vi "PPG_ABCGUI.panel.vi"() -> ()   [LabVIEW 2014, in "PPG_ABCGUI.lvlib"]
doc: "GUI to configure the FPGA card\n\nauthor: Dennis Neidherr, GSI\nlicense: GPL"
uses:
  PPG_ABCGUI.lvlib
  CSlibraries-extern/DimLVEvent/DimIndicators/DimIndicators.numericType.ctl
  CSlibraries-extern/DimLVEvent/DimIndicators/DimIndicators.anyType.ctl
  <vilib>/Utility/config.llb/Write Key (String).vi
  <vilib>/Utility/config.llb/Read Key (String).vi
  CSCore/CSSystem/CoreLib/CoreLib.int 2 byte array.vi
  CSCore/CSSystem/CoreLib/CoreLib.string 2 byte array.vi
  CSCore/CSSystem/CoreLib/CoreLib.double array 2 byte array.vi
  CSCore/CSSystem/CoreLib/CoreLib.lvlib
  CSCore/CSObj/CSObj.lvlib
  CSlibraries/UtilityLib/UtilityLib.lvlib
  CSCore/GUIs/GOGUserGUIs/DeviceBaseGUI/DeviceBaseGUI.lvlib
  CSlibraries-extern/DimLVEvent/DimIndicators/DimIndicators.lvlib
  CSCore/CSApplicationBaseClasses/DeviceBase/DeviceBase.lvlib
  CSCore/BaseProcess/BaseProcess.lvlib
  <vilib>/Utility/config.llb/NI_LVConfig.lvlib
panel:
  in  "Start":bool
  in  "SaveABC to File":bool
  in  "LoadABC from File":bool
  in  "LoadABC":bool
  out "FPGA state string":string
  in  "FPGA state":T1 caption="dic_service_numeric"
  in  "Outputs":string[][](table)
  in  "Timing":string[][](table)=[[""]]
  out "Busy":bool
  out "ErrorString":string
  out "deviceIDString":string
  out "loop counter":i32
  out "error out":errorcluster
  in  "error in (no error)":errorcluster
  in  "object ref":refnum<vi>
  in  "state":T1 caption="dic_service_numeric"
  in  "deviceID":T2 caption="dic_service_anyType"
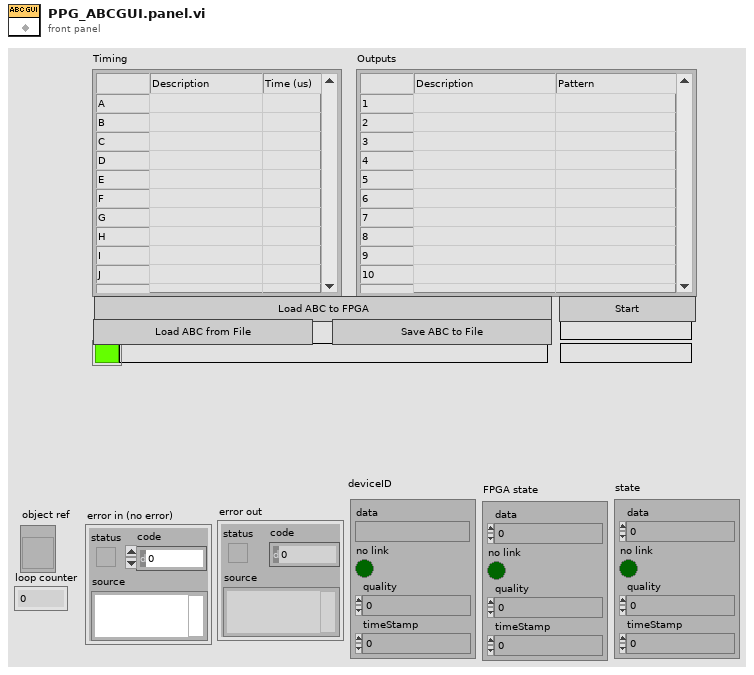
[diagram p1: front panel]
types:
  T1 = typedef "DimIndicators.lvlib/DimIndicators.numericType.ctl" = cluster{"data":dbl, "no link":bool, "quality":i32, "timeStamp":dbl}
  T2 = typedef "DimIndicators.lvlib/DimIndicators.anyType.ctl" = cluster{"data":string, "no link":bool, "quality":i32, "timeStamp":dbl}
  T3 = typedef "DeviceBaseGUI.lvlib/DeviceBaseGUI.i attribute.ctl" = cluster{"GOGFrontPanel.i attribute":T4}
  T4 = typedef "GOGFrontPanel.lvlib/GOGFrontPanel.i attribute.ctl" = cluster{"GOGObject":string, "Object":string, "Method":string, "Descriptor":T5, "Input Descriptor":string, "Output Descriptor":string, "inputNames":string[], "outputNames":string[], "Values":cluster{"descriptor":string, "value":string}[]}
  T5 = typedef "BaseProcess.lvlib/BaseProcess.descriptor string definition.ctl" = string
  T6 = enum8{"Enabled", "Disabled", "Disabled and Grayed Out"}
  T7 = typedef "CoreDefs.rawDataType.ctl" = i8[]
  T8 = typedef "NI_LVConfig.lvlib/Config Data RefNum.ctl" = refnum<k1>
  T9 = typedef "UtilityLib.lvlib/UtilityLib.valueStatus.ctl" = enum16{"no info available", "stand by/off", "on", "warning", "alarm/malfunction", "not implemented", "user action required", "important information", "system default", "control default", "indicator default", "button default"}
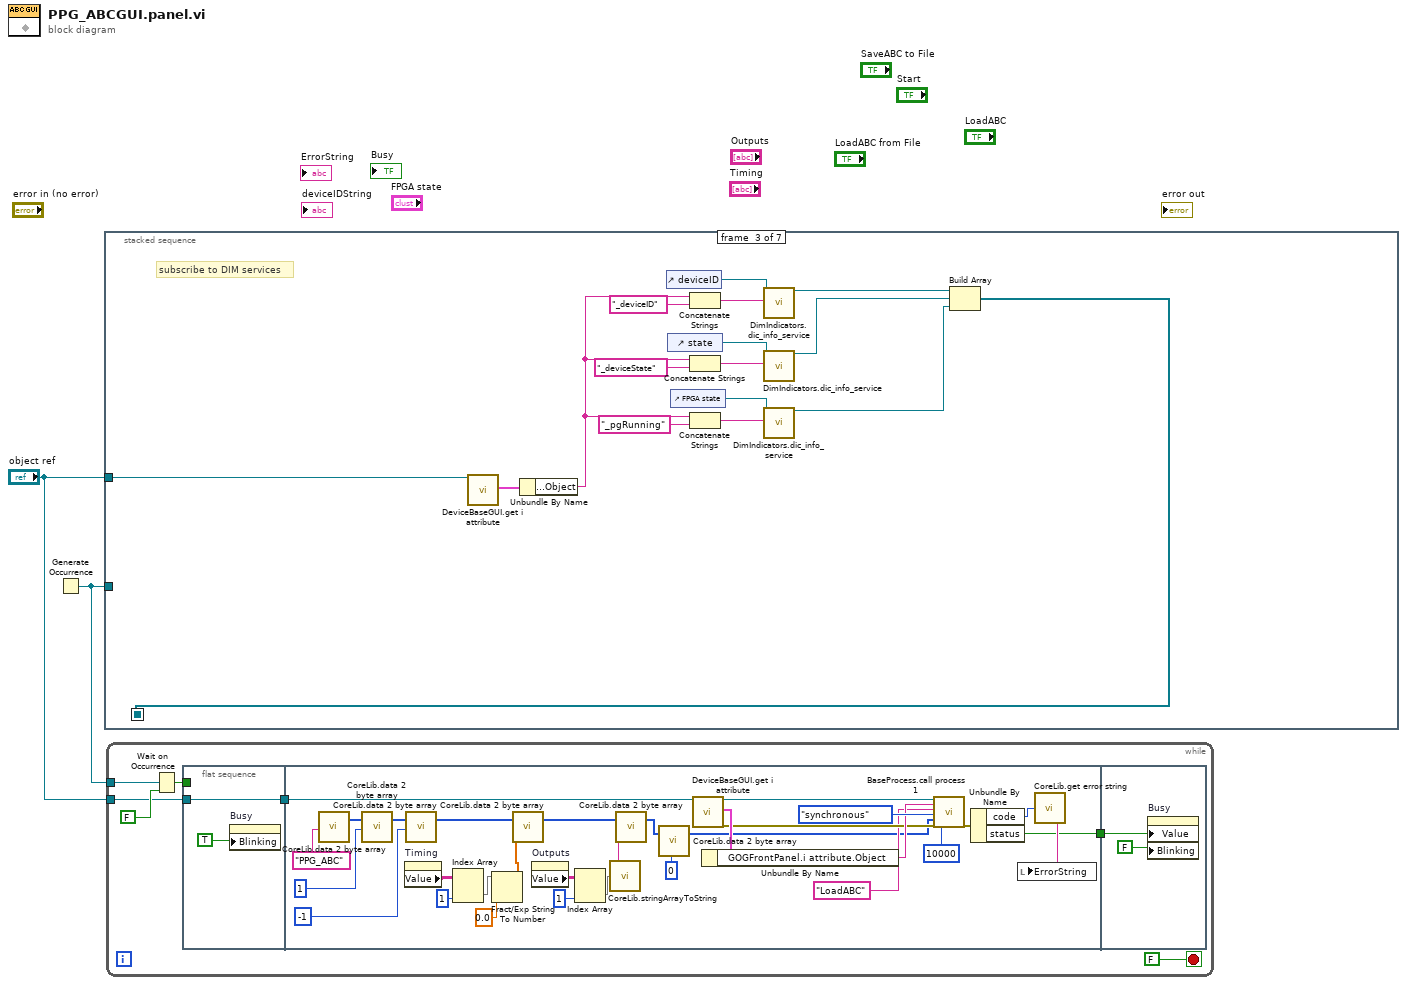
[diagram p0: block diagram]
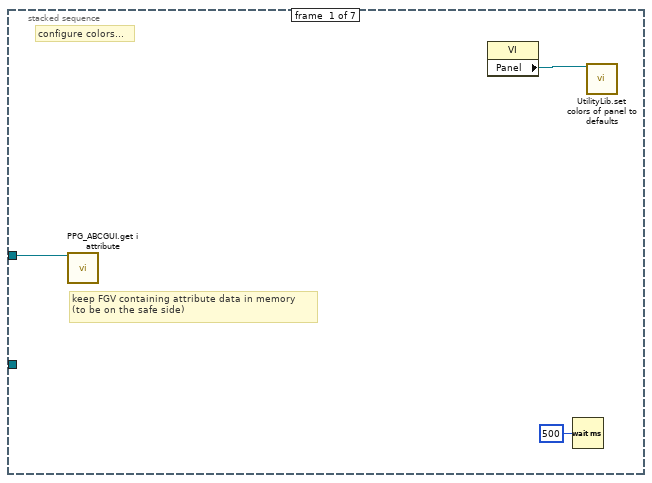
[diagram p2: hidden frame]
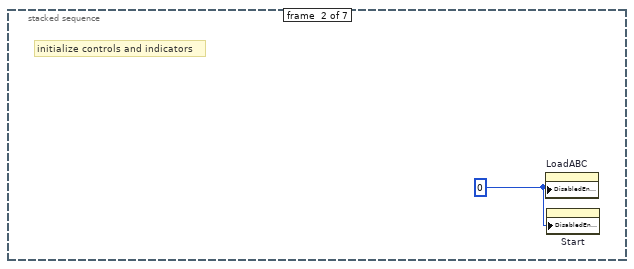
[diagram p3: hidden frame]
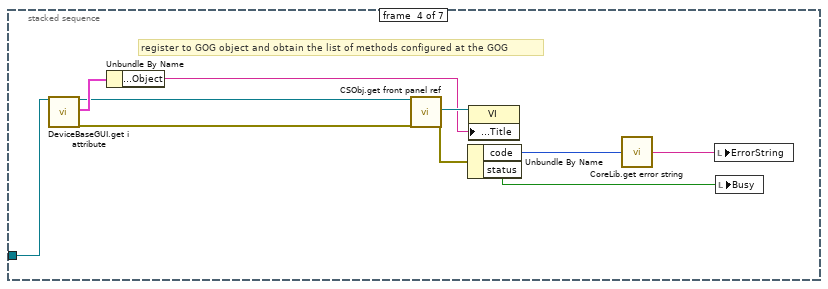
[diagram p4: hidden frame]
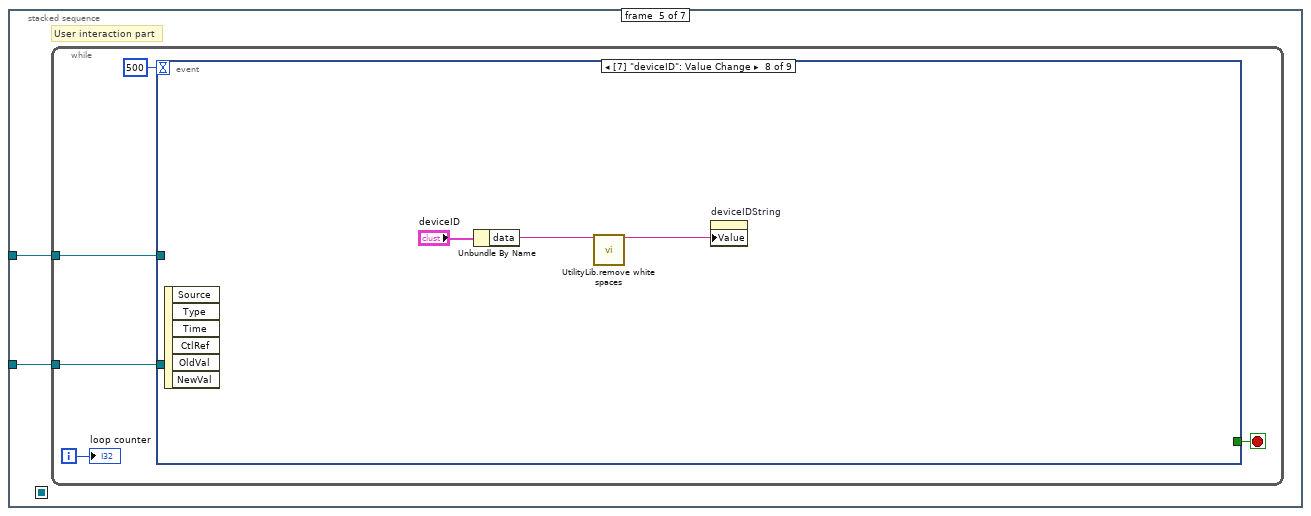
[diagram p5: hidden frame]
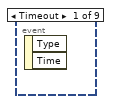
[diagram p6: hidden frame]
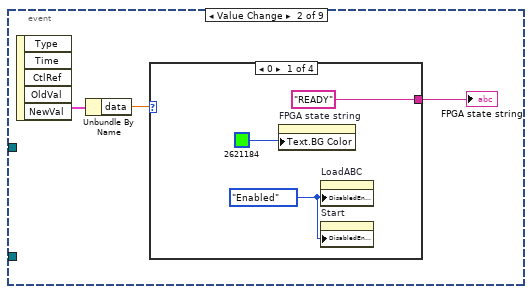
[diagram p7: hidden frame]
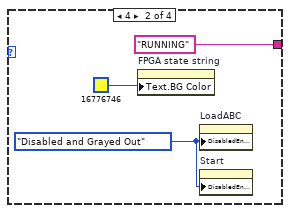
[diagram p8: hidden frame]
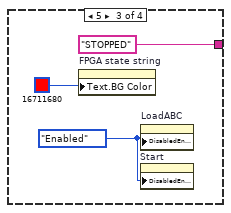
[diagram p9: hidden frame]
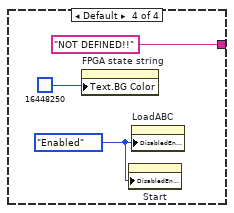
[diagram p10: hidden frame]
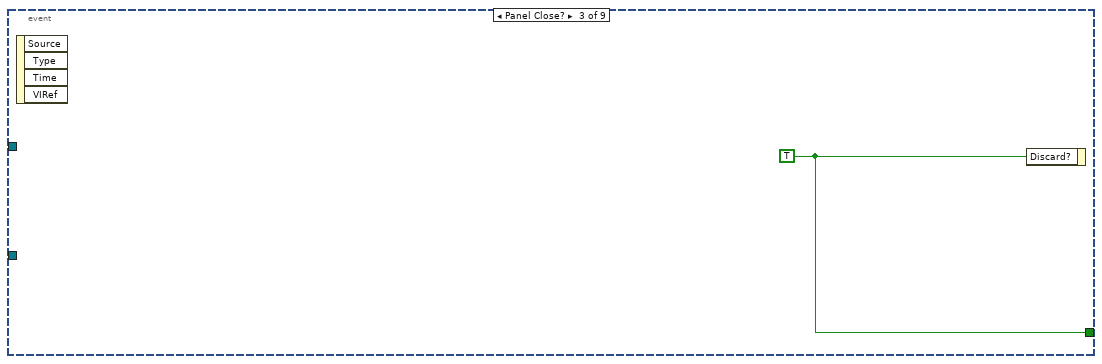
[diagram p11: hidden frame]
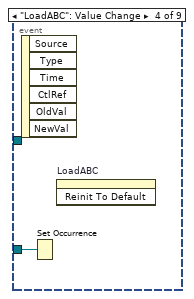
[diagram p12: hidden frame]
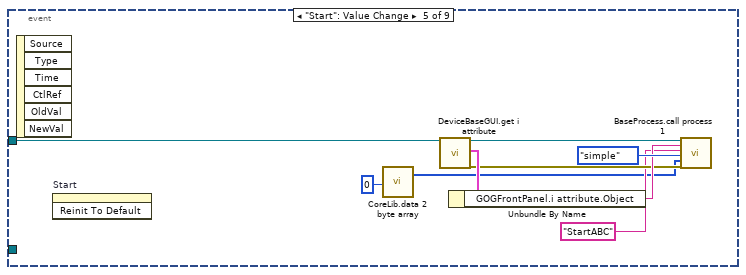
[diagram p13: hidden frame]
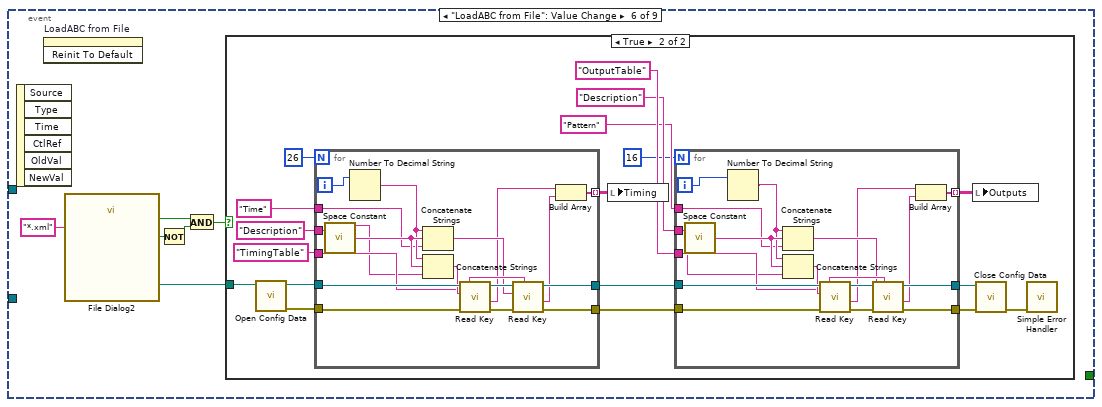
[diagram p14: hidden frame]
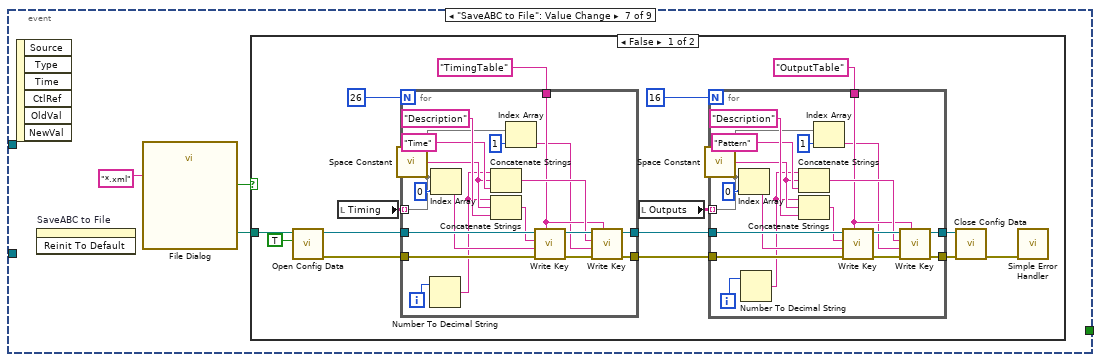
[diagram p16: hidden frame]
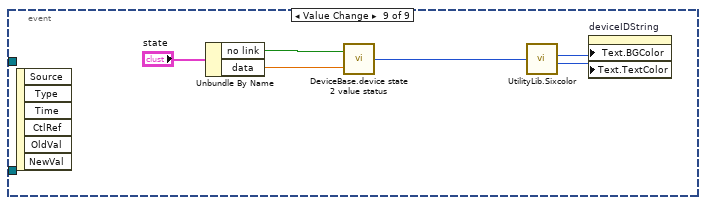
[diagram p18: hidden frame]
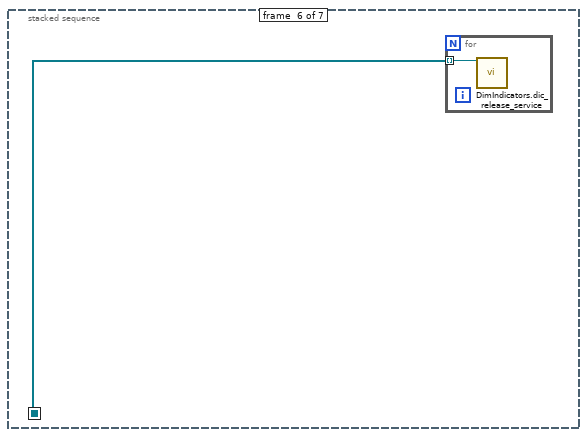
[diagram p19: hidden frame]
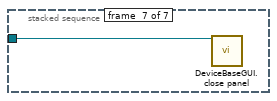
[diagram p20: hidden frame]
diagram:
  n1 = Generate Occurrence() -> (w1:refnum<k4>)
  n2 = stacked-sequence {
    seq-local: [_ _ w12 _ _ _ _] -> [_ _ _ _ _ w189 _]
    tunnel: "object ref" -> [w3 _ w22 w32 w34 _ w191]
    tunnel: w1 -> [_ _ _ _ w33 _ _]
    frame #0 {
      # "keep FGV containing attribute data in memory\n(to be on the safe side)"
      # "configure colors..."
      n3 = call "PPG_ABCGUI.get i attribute.vi"("i ref in"=w3) -> ()  [unwired: 16 in, 3 out]
      n4 = property class="VI"() -> ("Panel"=w4:refnum<vi>)  [unwired: 2 in, 2 out]
      n5 = Wait (ms)(milliseconds to wait=u32 500) -> ()  [unwired: 1 out]
      n6 = call "UtilityLib.set colors of panel to defaults.vi"("Front Panel"=w4) -> ()  [unwired: 18 in, 1 out]
    }
    frame #1 {
      w6 = u8 0 ("Disabled")
      # "initialize controls and indicators"
      n7 = property on="LoadABC" class="Bool"("DisabledEnum"=w6) -> ()  [unwired: 2 in, 2 out]
      n8 = property on="Start" class="Bool"("DisabledEnum"=w6) -> ()  [unwired: 2 in, 2 out]
    }
    frame #2 {
      # "subscribe to DIM services"
      n9 = call "DeviceBaseGUI.get i attribute.vi"("i ref in"=w22) -> ("i attribute"=w21:T3)  [unwired: 16 in, 2 out]
      n10 = Unbundle By Name(w21) -> ("GOGFrontPanel.i attribute.Object"=w8:string)
      n11 = control-ref of="deviceID"() -> (w17:refnum<vi>)
      n12 = control-ref of="state"() -> (w15:refnum<vi>)
      n13 = control-ref of="FPGA state"() -> (w7:refnum<vi>)
      n14 = Concatenate Strings(w8, "_deviceID" ("string")) -> (w18:string)
      n15 = Concatenate Strings(w8, "_deviceState" ("string")) -> (w16:string)
      n16 = Concatenate Strings(w8, "_pgRunning" ("string")) -> (w9:string)
      n17 = call "DimIndicators.dic_info_service.vi"("controlRef"=w17, "serviceName"=w18) -> ("controlRef out"=w14:refnum<vi>)  [unwired: 16 in, 1 out]
      n18 = call "DimIndicators.dic_info_service.vi"("controlRef"=w15, "serviceName"=w16) -> ("controlRef out"=w13:refnum<vi>)  [unwired: 16 in, 1 out]
      n19 = call "DimIndicators.dic_info_service.vi"("controlRef"=w7, "serviceName"=w9) -> ("controlRef out"=w11:refnum<vi>)  [unwired: 16 in, 1 out]
      n20 = Build Array(w14, w13, w11) -> (w12:refnum<vi>[])
    }
    frame #3 {
      # "register to GOG object and obtain the list of methods configured at the GOG"
      n21 = call "DeviceBaseGUI.get i attribute.vi"("i ref in"=w32) -> ("i ref out"=w24:refnum<vi>, "i attribute"=w31:T3, "error out"=w23:errorcluster)  [unwired: 16 in]
      n22 = Unbundle By Name(w31) -> ("GOGFrontPanel.i attribute.Object"=w29:string)
      n23 = call "CSObj.get front panel ref.vi"("i ref in"=w24, "error in (no error)"=w23) -> ("frontPanelRef"=w30:refnum<vi>, "error out"=w25:errorcluster)  [unwired: 15 in, 1 out]
      n24 = Unbundle By Name(w25) -> ("code"=w28:i32, "status"=w26:bool)
      n25 = property class="VI"(reference=w30, "Front Panel Window:Title"=w29) -> ()  [unwired: 1 in, 2 out]
      n26 = call "CoreLib.get error string.vi"("Error Code"=w28) -> ("Error String"=w27:string)
      n27 = local write "ErrorString"(w27) -> ()
      n28 = local write "Busy"(w26) -> ()
    }
    frame #4 {
      # "User interaction part"
      n29 = while {
        tunnel: w34 -> [w38]
        tunnel: w33 -> [w36]
        i -> [w39]
        stop <- w35 stop-if-true
        n30 = event shown="[7] \"deviceID\": Value Change" {
          selector: _ -> [_ _ _ _ _ _ _ _ _]
          dyn-events: _ -> [_ _ _ _ _ _ _ _ _]
          timeout: 500 -> [_ _ _ _ _ _ _ _ _]
          tunnel: w38 -> [_ _ _ _ w59 _ _ _ _]
          tunnel: w36 -> [_ _ _ w56 _ _ _ _ _]
          tunnel: [_ _ w55 _ _ _ _ _ _] -> w35
          event Timeout {
            n31 = event-data() -> ()  [unwired: 1 in, 2 out]
          }
          event Value Change {
            n32 = event-data() -> ("NewVal"=w42:T1)  [unwired: 1 in, 4 out]
            n33 = Unbundle By Name(w42) -> ("data"=w41:dbl)
            n34 = case shown="0" w41 {
              tunnel: ["READY" ("FPGA state string") "RUNNING" ("FPGA state string") "STOPPED" ("FPGA state string") "NOT DEFINED!!" ("FPGA state string")] -> w40
              frame 0 {
                w43 = T6."Enabled" ("Disabled")
                n35 = property on="FPGA state string" class="Str"("Text.BG Color"=u32 2621184) -> ()  [unwired: 2 in, 2 out]
                n36 = property on="LoadABC" class="Bool"("DisabledEnum"=w43) -> ()  [unwired: 2 in, 2 out]
                n37 = property on="Start" class="Bool"("DisabledEnum"=w43) -> ()  [unwired: 2 in, 2 out]
              }
              frame 4 {
                w46 = T6."Disabled and Grayed Out" ("Disabled")
                n38 = property on="FPGA state string" class="Str"("Text.BG Color"=u32 16776746) -> ()  [unwired: 2 in, 2 out]
                n39 = property on="LoadABC" class="Bool"("DisabledEnum"=w46) -> ()  [unwired: 2 in, 2 out]
                n40 = property on="Start" class="Bool"("DisabledEnum"=w46) -> ()  [unwired: 2 in, 2 out]
              }
              frame 5 {
                w49 = T6."Enabled" ("Disabled")
                n41 = property on="FPGA state string" class="Str"("Text.BG Color"=u32 16711680) -> ()  [unwired: 2 in, 2 out]
                n42 = property on="LoadABC" class="Bool"("DisabledEnum"=w49) -> ()  [unwired: 2 in, 2 out]
                n43 = property on="Start" class="Bool"("DisabledEnum"=w49) -> ()  [unwired: 2 in, 2 out]
              }
              frame Default {
                w52 = T6."Enabled" ("Disabled")
                n44 = property on="FPGA state string" class="Str"("Text.BG Color"=u32 16448250) -> ()  [unwired: 2 in, 2 out]
                n45 = property on="Start" class="Bool"("DisabledEnum"=w52) -> ()  [unwired: 2 in, 2 out]
                n46 = property on="LoadABC" class="Bool"("DisabledEnum"=w52) -> ()  [unwired: 2 in, 2 out]
              }
            }
            "FPGA state string" <- w40
          }
          event Panel Close? {
            w55 = TRUE ("Discard?")
            n47 = event-data() -> ()  [unwired: 1 in, 4 out]
            n48 = event-data("Discard?"=w55) -> ()  [unwired: 1 in, 1 out]
          }
          event "LoadABC": Value Change {
            n49 = event-data() -> ()  [unwired: 1 in, 6 out]
            n50 = Set Occurrence(w56) -> ()
            n51 = invoke on="LoadABC" class="Bool" method="Reinit To Default"() -> ()  [unwired: 3 in, 3 out]
          }
          event "Start": Value Change {
            n52 = event-data() -> ()  [unwired: 1 in, 6 out]
            n53 = invoke on="Start" class="Bool" method="Reinit To Default"() -> ()  [unwired: 3 in, 3 out]
            n54 = call-poly "CoreLib.data 2 byte array.vi"("i32"=0) -> ("byteArray out"=w58:T7)  [unwired: 18 in]
            n55 = call "DeviceBaseGUI.get i attribute.vi"("i ref in"=w59) -> ("i ref out"=w64:refnum<vi>, "i attribute"=w63:T3, "error out"=w61:errorcluster)  [unwired: 16 in]
            n56 = Unbundle By Name(w63) -> ("GOGFrontPanel.i attribute.Object"=w62:string)
            n57 = call "BaseProcess.call process 1.vi"("i ref in"=w64, "Object"=w62, "Selector"="StartABC", "CallType"=enum16{"simple", "synchronous", "asynchronous"}."simple", "Data"=w58, "error in (no error)"=w61) -> ()  [unwired: 11 in, 3 out]
          }
          event "LoadABC from File": Value Change {
            n58 = event-data() -> ()  [unwired: 1 in, 6 out]
            n59 = invoke on="LoadABC from File" class="Bool" method="Reinit To Default"() -> ()  [unwired: 3 in, 3 out]
            n60 = call "File Dialog2"("pattern (all files)"="*.xml") -> ("selected path"=w71:path, "exists"=w67:bool, "cancelled"=w69:bool)  [unwired: 11 in, 1 out]
            n61 = Not(x=w69) -> (.not. x?=w68:bool)
            n62 = And(x=w67, y=w68) -> (x .and. y?=w66:bool)
            n63 = case shown="True" w66 {
              tunnel: w71 -> [_ w89]
              frame False {
              }
              frame True {
                n64 = call <vilib>:"Open Config Data.vi"("configuration file path"=w89) -> ("error out"=w88:errorcluster, "refnum"=w87:T8)  [unwired: 8 in, 1 out]
                n65 = for {
                  N: 26 -> [_]
                  tunnel: w88 -> [w122]
                  tunnel: w87 -> [w123]
                  tunnel: "TimingTable" ("section") -> [w117]
                  tunnel: "Description" ("string") -> [w108]
                  tunnel: "Time" ("string") -> [w107]
                  tunnel: [w115] -> w81
                  tunnel: [w114] -> w80
                  tunnel: [w111] -> w82 mode=indexing
                  i -> [w110]
                  n66 = call <vilib>:"Space Constant.vi"() -> ("String"=w121:string)
                  n67 = Number To Decimal String(number=w110) -> (decimal integer string=w109:string)  [unwired: 1 in]
                  n68 = Concatenate Strings(w109, w121, w107) -> (w116:string)
                  n69 = Concatenate Strings(w109, w121, w108) -> (w120:string)
                  n70 = call-poly <vilib>:"Read Key.vi"("section"=w117, "error in (no error)"=w122, "key"=w120, "refnum"=w123) -> ("error out"=w119:errorcluster, "value"=w113:string, "refnum out"=w118:T8)  [unwired: 4 in, 1 out]
                  n71 = call-poly <vilib>:"Read Key.vi"("section"=w117, "error in (no error)"=w119, "key"=w116, "refnum"=w118) -> ("error out"=w115:errorcluster, "value"=w112:string, "refnum out"=w114:T8)  [unwired: 4 in, 1 out]
                  n72 = Build Array(w113, w112) -> (w111:string[])
                }
                n73 = local write "Timing"(w82) -> ()
                n74 = for {
                  N: 16 -> [_]
                  tunnel: w81 -> [w105]
                  tunnel: w80 -> [w106]
                  tunnel: "OutputTable" ("section") -> [w100]
                  tunnel: "Description" ("string") -> [w91]
                  tunnel: "Pattern" ("string") -> [w90]
                  tunnel: [w98] -> w73
                  tunnel: [w97] -> w74
                  tunnel: [w94] -> w75 mode=indexing
                  i -> [w93]
                  n75 = call <vilib>:"Space Constant.vi"() -> ("String"=w104:string)
                  n76 = Number To Decimal String(number=w93) -> (decimal integer string=w92:string)  [unwired: 1 in]
                  n77 = Concatenate Strings(w92, w104, w90) -> (w99:string)
                  n78 = Concatenate Strings(w92, w104, w91) -> (w103:string)
                  n79 = call-poly <vilib>:"Read Key.vi"("section"=w100, "error in (no error)"=w105, "key"=w103, "refnum"=w106) -> ("error out"=w102:errorcluster, "value"=w96:string, "refnum out"=w101:T8)  [unwired: 4 in, 1 out]
                  n80 = call-poly <vilib>:"Read Key.vi"("section"=w100, "error in (no error)"=w102, "key"=w99, "refnum"=w101) -> ("error out"=w98:errorcluster, "value"=w95:string, "refnum out"=w97:T8)  [unwired: 4 in, 1 out]
                  n81 = Build Array(w96, w95) -> (w94:string[])
                }
                n82 = local write "Outputs"(w75) -> ()
                n83 = call <vilib>:"Close Config Data.vi"("error in (no error)"=w73, "refnum"=w74) -> ("error out"=w72:errorcluster)  [unwired: 8 in, 1 out]
                n84 = call <vilib>:"Simple Error Handler.vi"("error in (no error)"=w72) -> ()  [unwired: 4 in, 5 out]
              }
            }
          }
          event "SaveABC to File": Value Change {
            n85 = event-data() -> ()  [unwired: 1 in, 6 out]
            n86 = invoke on="SaveABC to File" class="Bool" method="Reinit To Default"() -> ()  [unwired: 3 in, 3 out]
            n87 = call "File Dialog"("pattern (all files)"="*.xml") -> ("selected path"=w126:path, "cancelled"=w124:bool)  [unwired: 11 in, 2 out]
            n88 = case shown="False" w124 {
              tunnel: w126 -> [w141 _]
              frame False {
                n89 = call <vilib>:"Open Config Data.vi"("create file if necessary (T)"=TRUE, "configuration file path"=w141) -> ("error out"=w139:errorcluster, "refnum"=w138:T8)  [unwired: 7 in, 1 out]
                n90 = local read "Timing"() -> (w135:string[][])
                n91 = for {
                  N: 26 -> [_]
                  tunnel: w139 -> [w179]
                  tunnel: w138 -> [w178]
                  tunnel: "TimingTable" ("section") -> [w168]
                  tunnel: w135 -> [w167] mode=indexing
                  tunnel: [w164] -> w134
                  tunnel: [w163] -> w133
                  i -> [w162]
                  n92 = call <vilib>:"Space Constant.vi"() -> ("String"=w171:string)
                  n93 = Number To Decimal String(number=w162) -> (decimal integer string=w161:string)  [unwired: 1 in]
                  n94 = Index Array(array=w167, index=0) -> (element=w174:string)
                  n95 = Concatenate Strings(w161, w171, "Time" ("string")) -> (w170:string)
                  n96 = Concatenate Strings(w161, w171, "Description" ("string")) -> (w176:string)
                  n97 = Index Array(array=w167, index=1) -> (element=w165:string)
                  n98 = call-poly <vilib>:"Write Key.vi"("section"=w168, "error in (no error)"=w179, "value"=w174, "key"=w176, "refnum"=w178) -> ("error out"=w169:errorcluster, "refnum out"=w173:T8)  [unwired: 4 in, 1 out]
                  n99 = call-poly <vilib>:"Write Key.vi"("section"=w168, "error in (no error)"=w169, "value"=w165, "key"=w170, "refnum"=w173) -> ("error out"=w164:errorcluster, "refnum out"=w163:T8)  [unwired: 4 in, 1 out]
                }
                n100 = local read "Outputs"() -> (w132:string[][])
                n101 = for {
                  N: 16 -> [_]
                  tunnel: w134 -> [w160]
                  tunnel: w133 -> [w159]
                  tunnel: "OutputTable" ("section") -> [w149]
                  tunnel: w132 -> [w148] mode=indexing
                  tunnel: [w145] -> w128
                  tunnel: [w144] -> w129
                  i -> [w143]
                  n102 = call <vilib>:"Space Constant.vi"() -> ("String"=w152:string)
                  n103 = Index Array(array=w148, index=0) -> (element=w155:string)
                  n104 = Number To Decimal String(number=w143) -> (decimal integer string=w142:string)  [unwired: 1 in]
                  n105 = Concatenate Strings(w142, w152, "Pattern" ("string")) -> (w151:string)
                  n106 = Concatenate Strings(w142, w152, "Description" ("string")) -> (w157:string)
                  n107 = Index Array(array=w148, index=1) -> (element=w146:string)
                  n108 = call-poly <vilib>:"Write Key.vi"("section"=w149, "error in (no error)"=w160, "value"=w155, "key"=w157, "refnum"=w159) -> ("error out"=w150:errorcluster, "refnum out"=w154:T8)  [unwired: 4 in, 1 out]
                  n109 = call-poly <vilib>:"Write Key.vi"("section"=w149, "error in (no error)"=w150, "value"=w146, "key"=w151, "refnum"=w154) -> ("error out"=w145:errorcluster, "refnum out"=w144:T8)  [unwired: 4 in, 1 out]
                }
                n110 = call <vilib>:"Close Config Data.vi"("error in (no error)"=w128, "refnum"=w129) -> ("error out"=w127:errorcluster)  [unwired: 8 in, 1 out]
                n111 = call <vilib>:"Simple Error Handler.vi"("error in (no error)"=w127) -> ()  [unwired: 4 in, 5 out]
              }
              frame True {
              }
            }
          }
          event Value Change {
            n112 = event-data() -> ()  [unwired: 1 in, 6 out]
            n113 = Unbundle By Name("deviceID") -> ("data"=w182:string)
            n114 = call "UtilityLib.remove white spaces.vi"("string with blanks"=w182) -> ("string without white spaces"=w181:string)  [unwired: 14 in, 4 out]
            n115 = property on="deviceIDString" class="Str"("Value"=w181) -> ()  [unwired: 2 in, 2 out]
          }
          event Value Change {
            n116 = event-data() -> ()  [unwired: 1 in, 6 out]
            n117 = Unbundle By Name("state") -> ("no link"=w188:bool, "data"=w185:dbl)
            n118 = call "DeviceBase.device state 2 value status.vi"("deviceState"=w185, "no link"=w188) -> ("valueStatus"=w187:T9)
            n119 = call "UtilityLib.Sixcolor.vi"("State"=w187) -> ("elementBackground"=w186:u32, "elementText"=w183:u32)  [unwired: 2 in, 2 out]
            n120 = property on="deviceIDString" class="Str"("Text.BGColor"=w186, "Text.TextColor"=w183) -> ()  [unwired: 2 in, 2 out]
          }
        }
        "loop counter" <- w39
      }
    }
    frame #5 {
      n121 = for {
        tunnel: w189 -> [w190] mode=indexing
        n122 = call "DimIndicators.dic_release_service.vi"("controlRef"=w190) -> ()  [unwired: 18 in, 1 out]
      }
    }
    frame #6 {
      n123 = call "DeviceBaseGUI.close panel.vi"("i ref in"=w191) -> ()  [unwired: 17 in, 2 out]
    }
  }
  n124 = while {
    tunnel: w1 -> [w196]
    tunnel: "object ref" -> [w193]
    stop <- FALSE stop-if-true
    n125 = Wait on Occurrence(1:FALSE ("ignore previous (T)"), 2:w196) -> (0:w195:bool)  [unwired: 1 in]
    n126 = flat-sequence {
      tunnel: w195 -> [_]
      tunnel: [w199] -> w194
      tunnel: w193 -> [w199]
      tunnel: w194 -> [w226]
      tunnel: [w229] -> w192
      tunnel: w192 -> [w232]
      frame #0 {
        n127 = property on="Busy" class="Bool (strict)"("Blinking"=TRUE) -> ()  [unwired: 2 in, 2 out]
      }
      frame #1 {
        n128 = call-poly "CoreLib.data 2 byte array.vi"("string"="PPG_ABC") -> ("byteArray out"=w218:T7)  [unwired: 18 in]
        n129 = call-poly "CoreLib.data 2 byte array.vi"("byteArray"=w218, "i32"=1) -> ("byteArray out"=w216:T7)  [unwired: 17 in]
        n130 = property on="Timing" class="Tbl (strict)"() -> ("Value"=w210:string[][])  [unwired: 2 in, 2 out]
        n131 = call-poly "CoreLib.data 2 byte array.vi"("byteArray"=w216, "i32"=-1) -> ("byteArray out"=w214:T7)  [unwired: 17 in]
        n132 = Index Array(array=w210, index (col)=1 ("disabled index (col)")) -> (element=w212:string[])  [unwired: 1 in]
        n133 = Fract/Exp String To Number(string=w212, default (0 dbl)=0.0 ("disabled index (col)")) -> (number=w209:dbl[])  [unwired: 2 in, 1 out]
        n134 = call-poly "CoreLib.data 2 byte array.vi"("byteArray"=w214, "[d64]"=w209) -> ("byteArray out"=w205:T7)  [unwired: 17 in]
        n135 = property on="Outputs" class="Tbl (strict)"() -> ("Value"=w206:string[][])  [unwired: 2 in, 2 out]
        n136 = Index Array(array=w206, index (col)=1 ("disabled index (col)")) -> (element=w208:string[])  [unwired: 1 in]
        n137 = call "CoreLib.stringArrayToString.vi"("Array"=w208) -> ("String"=w204:string)
        n138 = call-poly "CoreLib.data 2 byte array.vi"("byteArray"=w205, "string"=w204) -> ("byteArray out"=w203:T7)  [unwired: 17 in]
        n139 = call-poly "CoreLib.data 2 byte array.vi"("byteArray"=w203, "i32"=0) -> ("byteArray out"=w202:T7)  [unwired: 17 in]
        n140 = call "DeviceBaseGUI.get i attribute.vi"("i ref in"=w226) -> ("i ref out"=w225:refnum<vi>, "i attribute"=w224:T3, "error out"=w222:errorcluster)  [unwired: 16 in]
        n141 = Unbundle By Name(w224) -> ("GOGFrontPanel.i attribute.Object"=w223:string)
        n142 = call "BaseProcess.call process 1.vi"("i ref in"=w225, "Object"=w223, "Selector"="LoadABC", "CallType"=enum16{"simple", "synchronous", "asynchronous"}."synchronous", "Data"=w202, "error in (no error)"=w222, "timeout (ms)"=10000 ("ms timeout (100)")) -> ("error out"=w220:errorcluster)  [unwired: 10 in, 2 out]
        n143 = Unbundle By Name(w220) -> ("code"=w231:i32, "status"=w229:bool)
        n144 = call "CoreLib.get error string.vi"("Error Code"=w231) -> ("Error String"=w230:string)
        n145 = local write "ErrorString"(w230) -> ()
      }
      frame #2 {
        n146 = property on="Busy" class="Bool (strict)"("Value"=w232, "Blinking"=FALSE) -> ()  [unwired: 2 in, 2 out]
      }
    }
  }
